vi "Leaktest Clear Chart Hist v3.vi"(0 "Absolute Pres Cht Ref":refnum<vi>, 5 "Diff Pres Cht Ref":refnum<vi>, 7 "Temp Cht Ref":refnum<vi>, 9 "Heat % Cht ref":refnum<vi>, 11 "error in (no error)":errorcluster) -> (15 "error out":errorcluster)   [LabVIEW 2020]
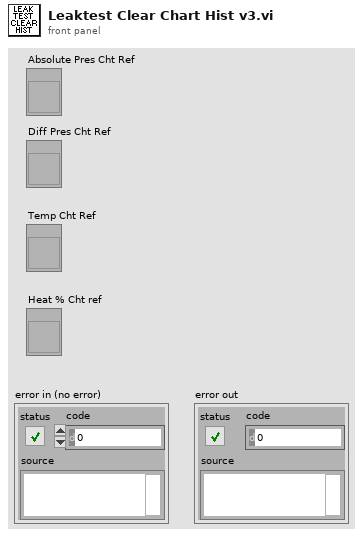
[diagram p1: front panel]
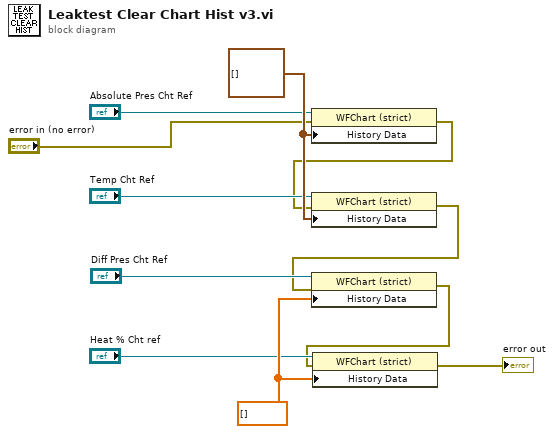
[diagram p0: block diagram]
diagram:
  w10 = dbl[] [] ("History Data")
  w11 = cluster{"Fill PSIA 1":dbl, "Fill PSIA 2":dbl}[] [] ("History Data")
  n1 = property class="WFChart (strict)"(reference="Absolute Pres Cht Ref", error in="error in (no error)", "History Data"=w11) -> (error out=w4:errorcluster)  [unwired: 1 out]
  n2 = property class="WFChart (strict)"(reference="Temp Cht Ref", error in=w4, "History Data"=w11) -> (error out=w3:errorcluster)  [unwired: 1 out]
  n3 = property class="WFChart (strict)"(reference="Diff Pres Cht Ref", error in=w3, "History Data"=w10) -> (error out=w2:errorcluster)  [unwired: 1 out]
  n4 = property class="WFChart (strict)"(reference="Heat % Cht ref", error in=w2, "History Data"=w10) -> (error out=→"error out":errorcluster)  [unwired: 1 out]
